vi "Convert Project Filenames.vi"(8 "Error In":errorcluster) -> (0 "Error Out":errorcluster)   [LabVIEW 2011]
panel:
  out "Array":path[](array[path])
  in  "Folder Path":path=path "/Macintosh HD/Users/Eric/labcode/LabVIEW/Maven/Maven PDL"
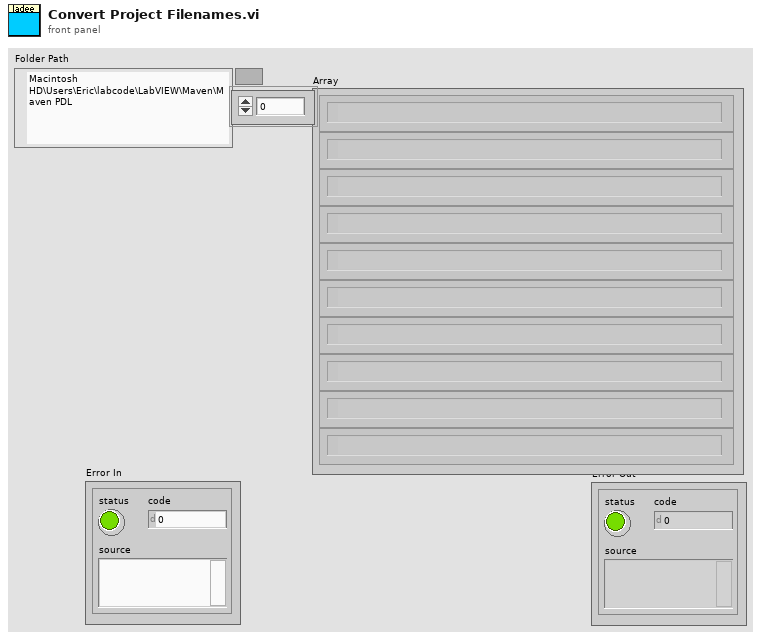
[diagram p1: front panel]
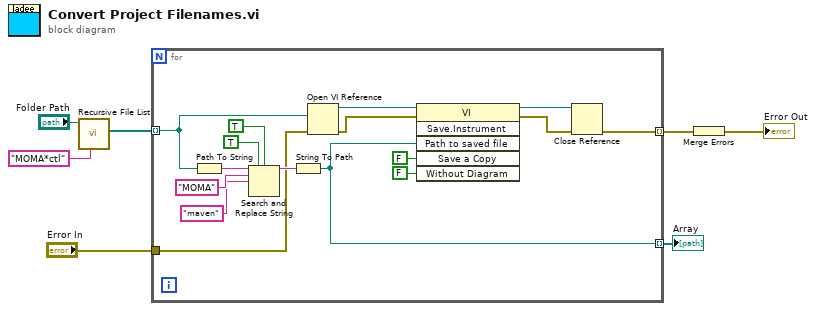
[diagram p0: block diagram]
diagram:
  n1 = call <vilib>:"Recursive File List.vi"("pattern"="MOMA*ctl", "Folder Path"="Folder Path") -> ("All Files in Dir"=w5:path[])  [unwired: 5 in, 4 out]
  n2 = for {
    tunnel: w5 -> [w22] mode=indexing
    tunnel: "Error In" -> [w13]
    tunnel: [w9] -> w3 mode=indexing
    tunnel: [w8] -> w1 mode=indexing
    n3 = Path To String(path=w22) -> (string=w21:string)
    n4 = Search and Replace String(replace all?=TRUE ("replace all? (F)"), case sensitive?=TRUE ("ignore case? (F)"), input string=w21, search string="MOMA", replace string="maven" ("replace string (\"\")")) -> (result string=w16:string)  [unwired: 3 in, 3 out]
    n5 = String To Path(string=w16) -> (path=w8:path)
    n6 = Open VI Reference(vi path=w22, error in (no error)=w13) -> (vi reference=w23:refnum<vi>, error out=w12:errorcluster)  [unwired: 4 in]
    n7 = invoke class="VI" method="Save.Instrument"(reference=w23, error in=w12, "Path to saved file"=w8, "Save a Copy"=FALSE, "Without Diagram"=FALSE) -> (reference out=w11:refnum<vi>, error out=w10:errorcluster)  [unwired: 1 in, 4 out]
    n8 = Close Reference(reference=w11, error in (no error)=w10) -> (error out=w9:errorcluster)
  }
  "Array" <- w1
  n9 = Merge Errors(w3) -> (→"Error Out":errorcluster)
